vi "Write EDR.vi"(10 "EDR":refnum<vi>, 11 "Main UI in":refnum<class "Main UI.lvclass">) -> (3 "Main UI out":refnum<class "Main UI.lvclass">)   [LabVIEW 2011, in "Main UI.lvclass"]
uses:
  Main UI.lvclass
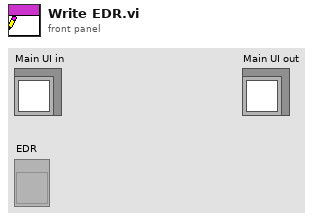
[diagram p1: front panel]
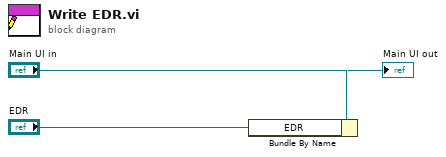
[diagram p0: block diagram]
diagram:
  n1 = Bundle By Name(cluster="Main UI in", "EDR"="EDR") -> (→"Main UI out":refnum<class "Main UI.lvclass">)
